vi "Is File a type of library.vi"(8 "error in (no error)":errorcluster, 11 "path":path) -> (0 "error out":errorcluster, 3 "Is library type?":bool)   [LabVIEW 2019, in "NI_FileType.lvlib"]
doc: "Returns TRUE if this file is a type of library, such as Libraries, XControls, XNodes, and LVClasses."
uses:
  NI_FileType.lvlib
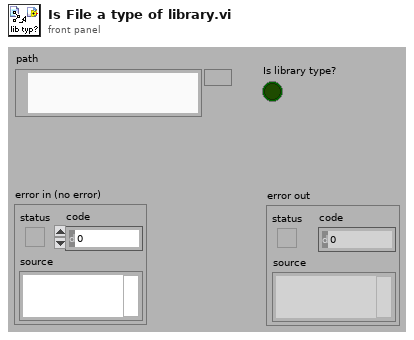
[diagram p1: front panel]
types:
  T1 = typedef "NI_FileType.lvlib/FT_FileTypes.ctl" = enum32{"Invalid file/path", "Unknown type", "Instrument", "Control", "Polymorphic VI", "Project", "Library", "LVClass", "XControl", "XNode", "CIN", "Run-time menu", "Palette menu", "LLB", "Shortcut", "Directory", "Class Private Data Control", "Statechart", "MathScript .m file", "Ladder Diagram", "LVLibp"}
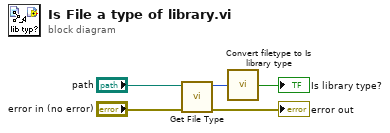
[diagram p0: block diagram]
diagram:
  n1 = call "Get File Type.vi"("error in (no error)"="error in (no error)", "path"="path") -> ("error out"=→"error out":errorcluster, "file type"=w2:T1)  [unwired: 7 in, 1 out]
  n2 = call "Convert filetype to Is library type.vi"("file type"=w2) -> ("Is library type?"=→"Is library type?":bool)  [unwired: 4 in]
